vi "Logic_Export_Raw_Digital_to_CSV.vi"(4 "error in (no error)":errorcluster, 5 "Enabled Digital Channels":i32[](array[numeric]), 6 "Filepath Input":string, 7 "Session Ref In":T1) -> (0 "error out":errorcluster, 1 "Debug Status":string, 3 "Session Ref Out":T1)   [LabVIEW 2023]
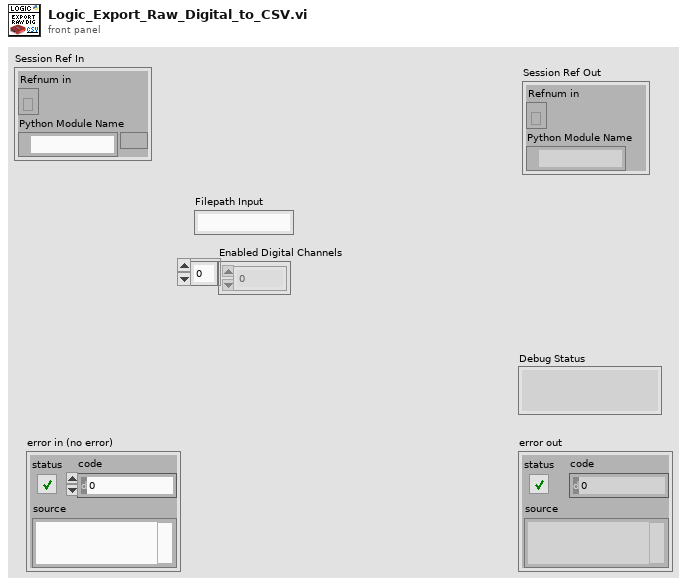
[diagram p1: front panel]
types:
  T1 = cluster{"Refnum in":refnum<k35>, "Python Module Name":path}
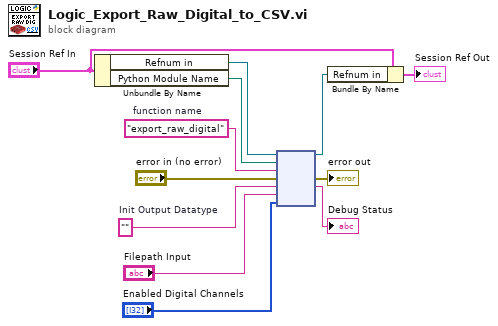
[diagram p0: block diagram]
diagram:
  w10 = "export_raw_digital"  # function name
  w9 = ""  # Init Output Datatype
  n1 = Unbundle By Name("Session Ref In") -> ("Refnum in"=w7:refnum<k35>, "Python Module Name"=w6:path)
  n2 = node(w7, w6, w10, "error in (no error)", w9, "Filepath Input", "Enabled Digital Channels") -> (w4:refnum<k35>, →"error out":errorcluster, →"Debug Status":string)  [unwired: 2 in, 2 out]
  n3 = Bundle By Name(cluster="Session Ref In", "Refnum in"=w4) -> (→"Session Ref Out":T1)
